vi "Prueba_Pt2Pt.vi"() -> ()   [LabVIEW 2017]
uses:
  <vilib>/ptbypt/NI_PtbyPt.lvlib
panel:
  out "Boolean 2":bool
  out "Boolean":bool
  in  "OK Button":bool
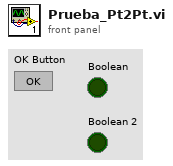
[diagram p1: front panel]
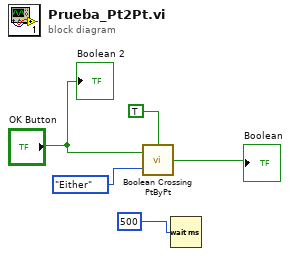
[diagram p0: block diagram]
diagram:
  n1 = call <vilib>:"Boolean Crossing PtByPt.vi"("initialize"=TRUE, "direction"=enum16{"Either", "F-T", "T-F"}."Either", "input"="OK Button") -> ("crossing"=→"Boolean":bool)
  n2 = Wait (ms)(milliseconds to wait=500) -> ()  [unwired: 1 out]
  "Boolean 2" <- "OK Button"
